vi "Is Null VVariant__ogtk.vi"(1 "Variant":variant) -> (0 "Null VVariant?":bool)   [LabVIEW 2023, in "openg_variant.lvlib"]
uses:
  openg_variant.lvlib
panel:
  # "EXPERIMENTAL"
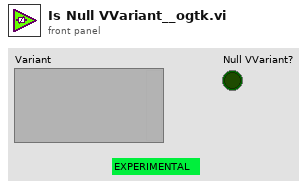
[diagram p1: front panel]
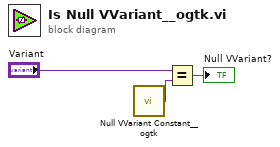
[diagram p0: block diagram]
diagram:
  n1 = call "Null VVariant Constant__ogtk.vi"() -> ("Null VVariant"=w2:variant)
  n2 = Equal?(x="Variant", y=w2) -> (x = y?=→"Null VVariant?":bool)
